vi "REM IO - Get Data Clusters.vi"(8 "error in (no error)":errorcluster, 9 "Output VS Refs":T5[](array[typedef]) format="%.0x", 10 "Input VS Refs":T5[](array[typedef]) format="%.0x") -> (0 "error out":errorcluster, 1 "I/O Output Data":T4 {"BD Refs"."Data Reference" format="%.0x"}, 2 "I/O Input Data":T1 {"BD Refs"."Data Reference" format="%.0x"})   [LabVIEW 2020, in "SEECD Engine.lvlib"]
uses:
  SEECD Engine.lvlib
  <vilib>/NI VeriStand/Custom Device API/Custom Device Item Ref.ctl
  Type Defs/Output Data.ctl
  <vilib>/NI VeriStand/Custom Device API/Block Data Reference.ctl
  <vilib>/NI VeriStand/Custom Device API/Data Reference.ctl
  Type Defs/Input Data.ctl
  Type Defs/Data Ref FGV Command.ctl
  <vilib>/NI VeriStand/Custom Device API/Data Access Type.ctl
  <vilib>/NI VeriStand/Custom Device API/Custom Device API.lvlib
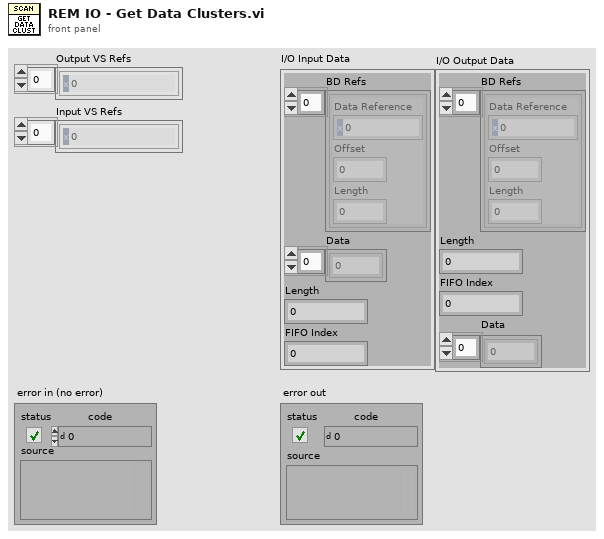
[diagram p1: front panel]
types:
  T1 = typedef "SEECD Engine.lvlib/Input Data.ctl" = cluster{"BD Refs":T2[], "Data":dbl[], "Length":i32, "FIFO Index":i32}
  T2 = typedef "Custom Device API.lvlib/Block Data Reference.ctl" = cluster{"Data Reference":T3, "Offset":u64, "Length":u64}
  T3 = typedef "Custom Device API.lvlib/Data Reference.ctl" = i32
  T4 = typedef "SEECD Engine.lvlib/Output Data.ctl" = cluster{"BD Refs":T2[], "Length":i32, "FIFO Index":i32, "Data":dbl[]}
  T5 = typedef "Custom Device API.lvlib/Custom Device Item Ref.ctl" = u64
  T6 = typedef "SEECD Engine.lvlib/Data Ref FGV Command.ctl" = enum16{"Intialize", "Get", "Update"}
  T7 = typedef "Custom Device API.lvlib/Data Access Type.ctl" = enum16{"Read", "Write"}
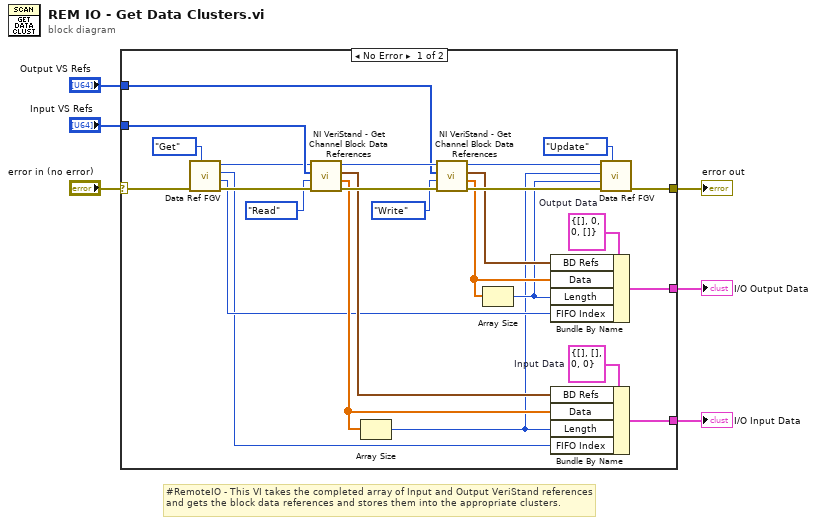
[diagram p0: block diagram]
diagram:
  # "#RemoteIO - This VI takes the completed array of Input and Output VeriStand references and gets the block data references and stores them into the appropriate clusters."
  n1 = case shown="No Error" "error in (no error)" {
    selector: "error in (no error)" -> [w31 w33]
    tunnel: "Input VS Refs" -> [w29 _]
    tunnel: "Output VS Refs" -> [w25 _]
    tunnel: [w19 w33] -> w3
    tunnel: [w12 _] -> w2
    tunnel: [w11 _] -> w1
    frame No Error {
      w18 = T4 {"BD Refs"=[], "Length"=0, "FIFO Index"=0, "Data"=[]}  # Output Data
      w17 = T1 {"BD Refs"=[], "Data"=[], "Length"=0, "FIFO Index"=0}  # Input Data
      n2 = call "Data Ref FGV.vi"("Command"=Data_Ref_FGV_Command."Get", "error in (no error)"=w31) -> ("error out"=w30:errorcluster, "Output FIFO Index / Length"=w9:i32, "Input FIFO Index / Length"=w7:i32, "Device Ref out"=w28:T5)  [unwired: 6 in]
      n3 = call <vilib>:"NI VeriStand - Get Channel Block Data References.vi"("error in (no error)"=w30, "Access"=Data_Access_Type."Read", "Channel Refs"=w29, "Device Ref in"=w28) -> ("error out"=w26:errorcluster, "Values Array"=w13:dbl[], "Block Data Refs"=w16:T2[], "Device Ref out"=w27:T5)  [unwired: 4 in]
      n4 = Array Size(array=w13) -> (size(s)=w8:i32)
      n5 = call <vilib>:"NI VeriStand - Get Channel Block Data References.vi"("error in (no error)"=w26, "Access"=Data_Access_Type."Write", "Channel Refs"=w25, "Device Ref in"=w27) -> ("error out"=w21:errorcluster, "Values Array"=w14:dbl[], "Block Data Refs"=w15:T2[], "Device Ref out"=w20:T5)  [unwired: 4 in]
      n6 = Array Size(array=w14) -> (size(s)=w10:i32)
      n7 = Bundle By Name(cluster=w18, "BD Refs"=w15, "Data"=w14, "Length"=w10, "FIFO Index"=w9) -> (w12:T4)
      n8 = Bundle By Name(cluster=w17, "BD Refs"=w16, "Data"=w13, "Length"=w8, "FIFO Index"=w7) -> (w11:T1)
      n9 = call "Data Ref FGV.vi"("Command"=Data_Ref_FGV_Command."Update", "error in (no error)"=w21, "Output Length"=w10, "Input Length"=w8, "Device Ref in"=w20) -> ("error out"=w19:errorcluster)  [unwired: 3 in, 3 out]
    }
    frame Error {
    }
  }
  "error out" <- w3
  "I/O Input Data" <- w1
  "I/O Output Data" <- w2
